vi "Get User_Access.vi"(8 "error in (no error)":errorcluster, 10 "GUID":string, 11 "Function in":refnum<class "Function.lvclass">) -> (0 "error out":errorcluster, 1 "found":bool, 2 "Connected Client Cluster":T2, 3 "Function out":refnum<class "Function.lvclass">, 4 "Access":T1)   [LabVIEW 2016, in "Function Actor.lvlib" / "Function.lvclass"]
uses:
  <userlib>/Common Components/Function Actor/Function.lvclass
  <userlib>/Common Components/Common/Connected Client Cluster.ctl
  <userlib>/Common Components/UserPwd DB/UserPwd DB/Access Level.ctl
  <userlib>/Common Components/Function Actor/Function.lvclass/Function.ctl
  <userlib>/Common Components/Common/Common.lvlib
  <userlib>/Common Components/UserPwd DB/UserPwd DB/UserPwd DB.lvclass
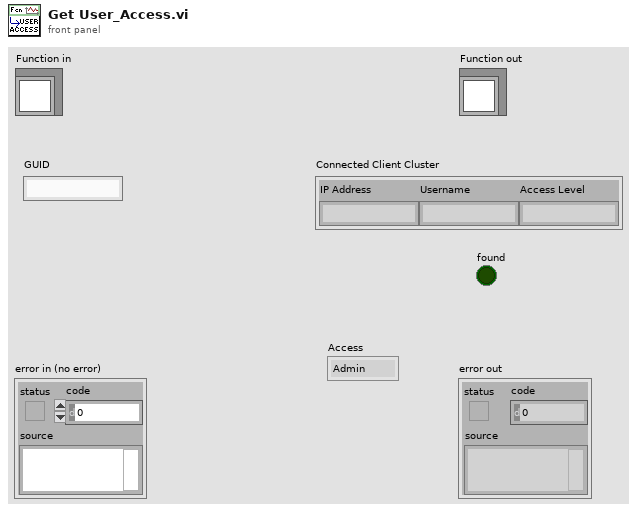
[diagram p1: front panel]
types:
  T1 = typedef "UserPwd DB.lvlib/UserPwd DB.lvclass/Access Level.ctl" = enum16{"Admin", "User lv1", "User lv2", "User lv3", "User lv4", "User lv5", "User lv6", "User lv7", "User lv8", "User lv9", "Guest"}
  T2 = typedef "Common.lvlib/Connected Client Cluster.ctl" = cluster{"IP Address":string, "Username":string, "Access Level":string}
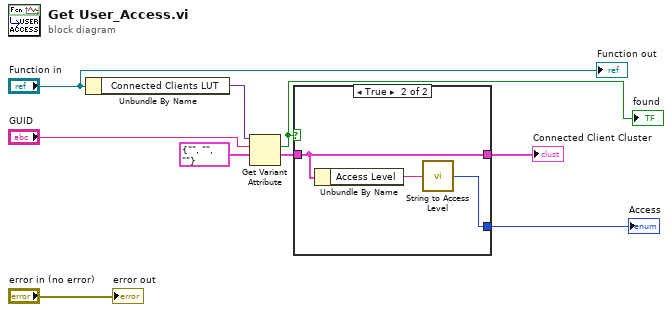
[diagram p0: block diagram]
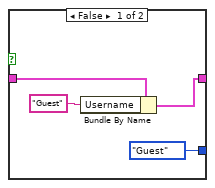
[diagram p2: hidden frame]
diagram:
  n1 = Unbundle By Name("Function in") -> ("Connected Clients LUT"=w7:variant)
  n2 = Get Variant Attribute(Variant=w7, name="GUID", default value (empty Variant)=T2 {"IP Address"="", "Username"="", "Access Level"=""} ("Connected Client Cluster")) -> (found=w4:bool, value=w3:T2)  [unwired: 1 in, 2 out]
  "found" <- w4
  n3 = case shown="True" w4 {
    tunnel: [w12 w15] -> w2
    tunnel: w3 -> [w13 w15]
    tunnel: [Access_Level."Guest" ("Access") w14] -> w1
    frame False {
      n4 = Bundle By Name(cluster=w13, "Username"="Guest") -> (w12:T2)
    }
    frame True {
      n5 = Unbundle By Name(w15) -> ("Access Level"=w16:string)
      n6 = call <userlib>:"String to Access Level.vi"("String"=w16) -> ("Access"=w14:T1)
    }
  }
  "Connected Client Cluster" <- w2
  "Access" <- w1
  "error out" <- "error in (no error)"
  "Function out" <- "Function in"
